vi "UI_Enable_Disable_Clusters.vi"(8 "error in (no error)":errorcluster, 10 "Enable ?":bool, 11 "Controls":refnum<vi>[](array[refnum])) -> (0 "error out":errorcluster caption="sortie d'erreur")   [LabVIEW 2018]
doc: "Définit toutes les commandes du tableau en entrée à la valeur \"État Activé\"."
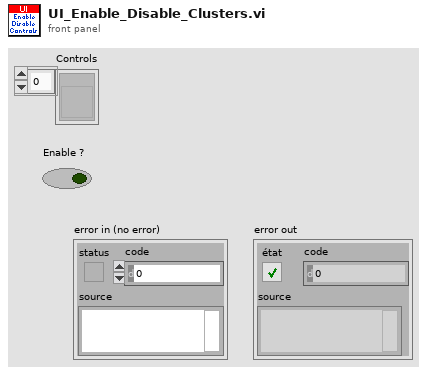
[diagram p1: front panel]
types:
  T1 = enum8{"Enabled", "Disabled", "Disabled and Grayed Out"}
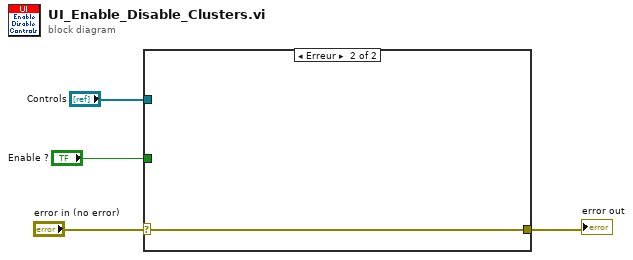
[diagram p0: block diagram]
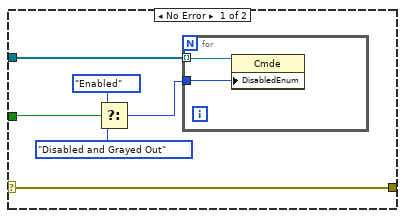
[diagram p2: hidden frame]
diagram:
  n1 = case shown="Erreur" "error in (no error)" {
    selector: "error in (no error)" -> [w5 w13]
    tunnel: "Controls" -> [w10 _]
    tunnel: "Enable ?" -> [w9 _]
    tunnel: [w5 w13] -> w1
    frame No Error {
      n2 = Select(t=T1."Enabled" ("Désactivé"), s=w9, f=T1."Disabled and Grayed Out" ("Désactivé")) -> (s? t:f=w8:T1)
      n3 = for {
        tunnel: w10 -> [w12] mode=indexing
        tunnel: w8 -> [w11]
        n4 = property class="Cmde"(reference=w12, "DisabledEnum"=w11) -> ()  [unwired: 1 in, 2 out]
      }
    }
    frame Error {
    }
  }
  "error out" <- w1
